vi "TestExec.HW Item List to Equipment List Table.vi"(3 "Equipment List":string[][](table)=[["", "", "", "", ""], ["", "", "", "", ""], ["", "", "", "", ""], ["", "", "", "", ""], ["", "", "", "", ""]], 11 "HW Items":T1[](array[typedef])) -> ()   [LabVIEW 2018]
uses:
  Common/Utils/Results/Result XML/TestResult.HW Item.ctl
panel:
  in  "Equipment List":refnum<vi>
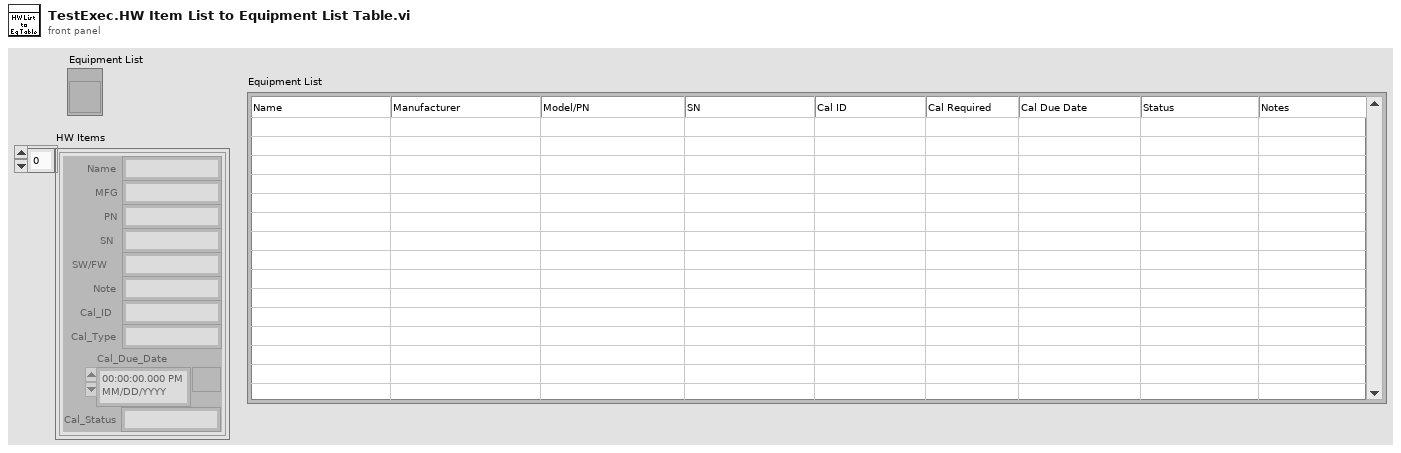
[diagram p1: front panel]
types:
  T1 = typedef "TestResult.HW Item.ctl" = cluster{"Name":string, "MFG":string, "PN":string, "SN":string, "SW/FW":string, "Note":string, "Cal_ID":string, "Cal_Type":string, "Cal_Due_Date":timestamp, "Cal_Status":string}
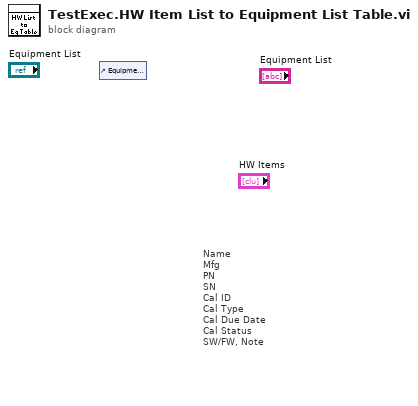
[diagram p0: block diagram]
diagram:
  # "Name\nMfg\nPN\nSN\nCal ID\nCal Type\nCal Due Date\nCal Status\nSW/FW, Note"
  n1 = control-ref of="Equipment List"() -> ()  [unwired: 1 out]
